vi "IterateShooter.vi"   [LabVIEW 2015]
uses:
  <vilib>/Rock Robotics/WPI/Solenoid/WPI_SolenoidValue.ctl
  <vilib>/Rock Robotics/WPI/Utilities/WPI_GetSetVariantRefNum.vi
  Robot Global Data.vi
  <vilib>/Rock Robotics/WPI/Solenoid/WPI_SolenoidSetEnum.vi
types:
  T1 = typedef "WPI_JoystickDevRef.ctl" = cluster{"Device":T2}
  T2 = typedef "WPI_JoystickDeviceEnum.ctl" = enum16{"USB 0", "USB 1", "USB 2", "USB 3", "USB 4", "USB 5"}
  T3 = typedef "constants.ctl" = cluster{"motorConstants":cluster{"leftDriveMotor":u8, "rightDriveMotor":u8, "climberWinch":T4, "shooterTopFlyWheel":T4, "shooterBottomFlyWheel":T4, "climberExtender":T4, "shooterIntakeWheel":u8, "Front Arm Motor":u8}, "arduinoInputChannel":cluster{"armAngleUp":i32, "intakeWheelSpinIn":i32, "winchUp":i32, "extenderUp":i32, "AimingAuto":i32, "extenderDown":i32, "FrontArmAxis":i32, "shooter up/down":i32}, "driveConstants":cluster{"firstIntervalPercent":dbl, "secondIntervalPercent":dbl, "thirdIntervalPercent":dbl}, "cRioInputChanels":cluster{"photoEye":i32, "limitExtender":i32}, "pneumaticsChannels":cluster{"angleSolenoid":T5, "shooterAnglerPneumaticForward":T5, "shooterAnglerPneumaticReverse":T5, "Pneumatics Control Module":u8}, "flyWheelConstants":cluster{"manualTopWheel":dbl, "manualBottomWheel":dbl, "autoFuncConst1":dbl, "autoFuncConst2":dbl, "autoFuncConst3":dbl, "autoFuncConst4":dbl, "Array":dbl[][]}}
  T4 = typedef "FPGA_DIOPWMChannel.ctl" = enum8{"PWM 0", "PWM 1", "PWM 2", "PWM 3", "PWM 4", "PWM 5", "PWM 6", "PWM 7", "PWM 8", "PWM 9", "PWM MXP 0", "PWM MXP 1", "PWM MXP 2", "PWM MXP 3", "PWM MXP 4", "PWM MXP 5", "PWM MXP 6", "PWM MXP 7", "PWM MXP 8", "PWM MXP 9", "Invalid"}
  T5 = typedef "WPI_SolenoidChannel.ctl" = enum8{"Solenoid 0", "Solenoid 1", "Solenoid 2", "Solenoid 3", "Solenoid 4", "Solenoid 5", "Solenoid 6", "Solenoid 7", "Invalid"}
  T6 = cluster{"Distance (ft)":dbl, "Center":cluster{dbl, dbl}, "Normalized Rect":cluster{"Numeric":dbl, "Numeric 2":dbl, "Numeric 3":dbl, "Numeric 5":dbl}}[]
  T7 = typedef "WPI_SolenoidValue.ctl" = enum16{"Off", "On", "Forward", "Reverse"}
  T8 = typedef "WPI_SolenoidDevRef.ctl" = cluster{"DevStatus":errorcluster, "Pneumatics Control Module":u8, "Forward Solenoid Channel":T5, "Reverse Solenoid Channel":T5}
  T9 = typedef "WPI_MotorControlDeviceRef.ctl" = cluster{"DeviceStatus":errorcluster, "Type":T10, "PWM":cluster{"PWM Channel":T4, "DeadBand":T11}, "CAN":cluster{"Device Number":u8, "Control Mode":T12, "Semaphore":T13, "Max Vout":dbl, "TalonSRX Control Mode":T14}, "Invert":bool}
  T10 = typedef "WPI_MotorControlType.ctl" = enum16{"PWM", "CAN", "CANTalonSRX"}
  T11 = typedef "WPI_PWMDeadband.ctl" = cluster{"Name":string, "maxPositivePwm":i32, "minPositivePwm":i32, "centerPwm":i32, "maxNegativePwm":i32, "minNegativePwm":i32, "angularRange":u16}
  T12 = typedef "WPI_CANJaguar_ControlMode.ctl" = enum8{"Percent VBus", "Current", "Speed", "Position", "Voltage"}
  T13 = typedef "Semaphore RefNum" = refnum<k1>
  T14 = typedef "WPI_CANTalonSRX_APIControlMode.ctl" = enum8{"Percent VBus", "Speed", "Position", "Slave", "Unchanged / Invalid", "Voltage Compensation", "Current", "Motion Profile"}
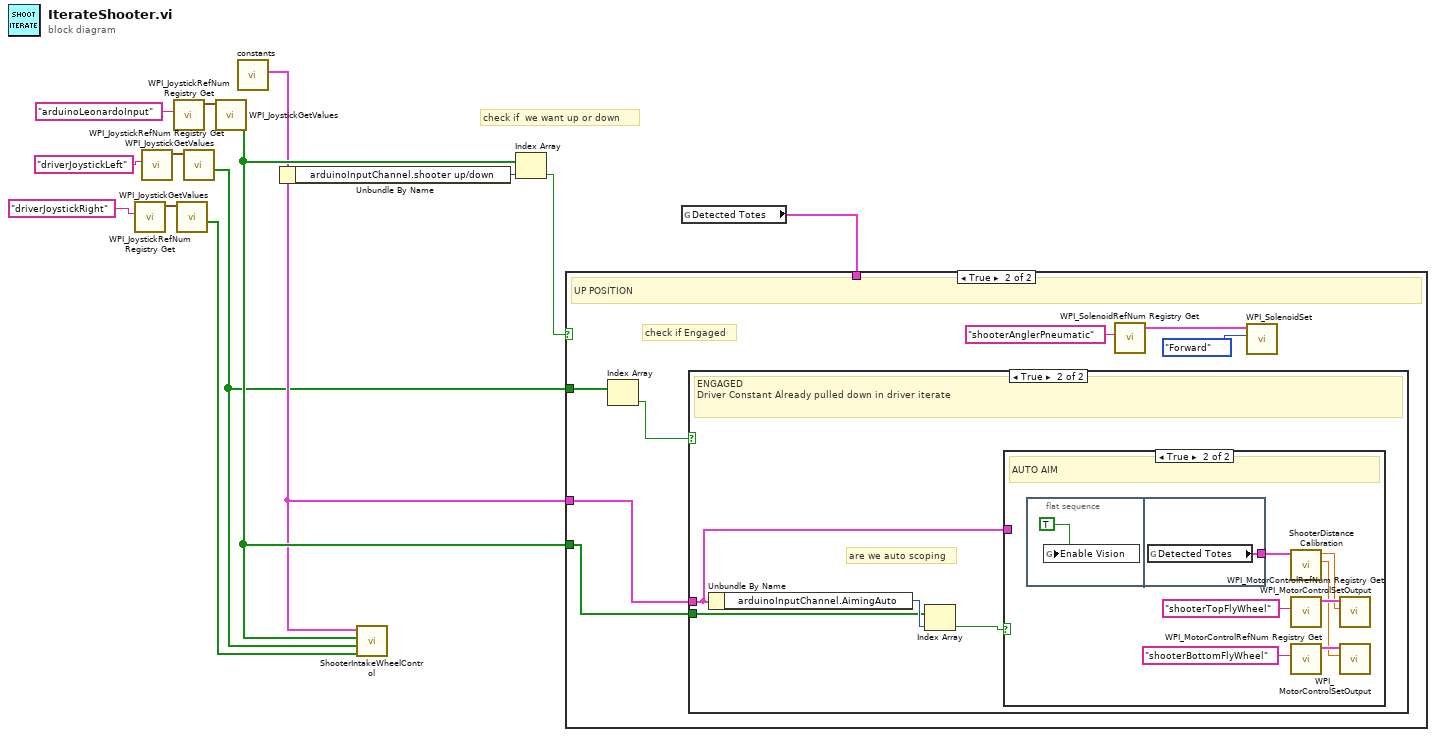
[diagram p0: block diagram]
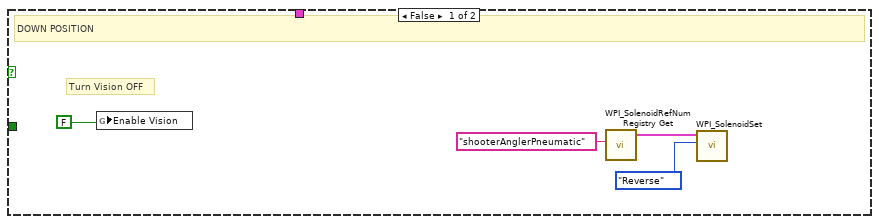
[diagram p2: hidden frame]
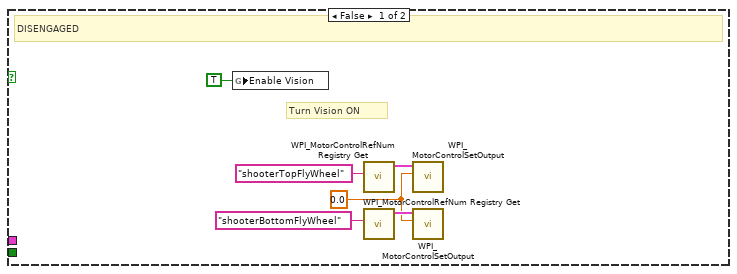
[diagram p3: hidden frame]
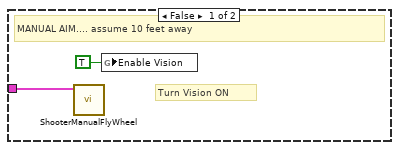
[diagram p4: hidden frame]
diagram:
  # "check if  we want up or down"
  n1 = call <vilib>:"WPI_JoystickRefNum Registry Get.vi"("refnum name"="driverJoystickRight") -> ("JoystickDevRef"=w8:T1)  [unwired: 9 in, 1 out]
  n2 = call <vilib>:"WPI_JoystickRefNum Registry Get.vi"("refnum name"="driverJoystickLeft") -> ("JoystickDevRef"=w9:T1)  [unwired: 9 in, 1 out]
  n3 = call <vilib>:"WPI_JoystickRefNum Registry Get.vi"("refnum name"="arduinoLeonardoInput") -> ("JoystickDevRef"=w12:T1)  [unwired: 9 in, 1 out]
  n4 = call <vilib>:"WPI_JoystickGetValues.vi"("JoystickDevRef"=w8) -> ("Buttons"=w4:bool[])  [unwired: 6 in, 4 out]
  n5 = call <vilib>:"WPI_JoystickGetValues.vi"("JoystickDevRef"=w9) -> ("Buttons"=w5:bool[])  [unwired: 6 in, 4 out]
  n6 = call <vilib>:"WPI_JoystickGetValues.vi"("JoystickDevRef"=w12) -> ("Buttons"=w7:bool[])  [unwired: 6 in, 4 out]
  n7 = call "constants.vi"() -> (2:w6:T3)  [unwired: 11 in]
  n8 = Unbundle By Name(w6) -> ("arduinoInputChannel.shooter up/down"=w11:i32)
  n9 = call "ShooterIntakeWheelControl.vi"("Constants"=w6, "leonardoJoystick"=w7, "driverJoystickLeft"=w5, "driverJoystickRight"=w4) -> ()  [unwired: 6 in]
  n10 = Index Array(array=w7, index=w11) -> (element=w10:bool)
  n11 = global read "Robot Global Data.vi" "Detected Totes"() -> (w1:T6)
  n12 = case shown="True" w10 {
    tunnel: w7 -> [_ w22]
    tunnel: w6 -> [_ w23]
    tunnel: w5 -> [_ w21]
    tunnel: w1 -> [_ _]
    frame False {
      # "Turn Vision OFF"
      # "DOWN POSITION"
      n13 = global write "Robot Global Data.vi" "Enable Vision"(FALSE ("Enable Vision")) -> ()
      n14 = call <vilib>:"WPI_SolenoidRefNum Registry Get.vi"("refnum name"="shooterAnglerPneumatic") -> ("SolenoidDevRef"=w15:T8)  [unwired: 9 in, 1 out]
      n15 = call-poly <vilib>:"WPI_SolenoidSet.vi"("Value"=WPI_SolenoidValue."Reverse", "SolenoidDevRef"=w15) -> ()  [unwired: 8 in, 2 out]
    }
    frame True {
      # "check if Engaged"
      # "UP POSITION"
      n16 = Index Array(array=w21) -> (element=w24:bool)  [unwired: 1 in]
      n17 = case shown="True" w24 {
        tunnel: w23 -> [_ w31]
        tunnel: w22 -> [_ w32]
        frame False {
          w26 = 0.0 ("Output")
          # "Turn Vision ON"
          # "DISENGAGED"
          n18 = global write "Robot Global Data.vi" "Enable Vision"(TRUE ("Enable Vision")) -> ()
          n19 = call <vilib>:"WPI_MotorControlRefNum Registry Get.vi"("refnum name"="shooterTopFlyWheel") -> ("MotorControlDevRef"=w25:T9)  [unwired: 9 in, 1 out]
          n20 = call <vilib>:"WPI_MotorControlRefNum Registry Get.vi"("refnum name"="shooterBottomFlyWheel") -> ("MotorControlDevRef"=w29:T9)  [unwired: 9 in, 1 out]
          n21 = call <vilib>:"WPI_MotorControlSetOutput.vi"("Output"=w26, "MotorControlDevRef"=w25) -> ()  [unwired: 7 in, 3 out]
          n22 = call <vilib>:"WPI_MotorControlSetOutput.vi"("Output"=w26, "MotorControlDevRef"=w29) -> ()  [unwired: 7 in, 3 out]
        }
        frame True {
          # "are we auto scoping"
          # "ENGAGED\nDriver Constant Already pulled down in driver iterate"
          n23 = Unbundle By Name(w31) -> ("arduinoInputChannel.AimingAuto"=w34:i32)
          n24 = Index Array(array=w32, index=w34) -> (element=w33:bool)
          n25 = case shown="True" w33 {
            tunnel: w31 -> [w35 _]
            frame False {
              # "Turn Vision ON"
              # "MANUAL AIM.... assume 10 feet away"
              n26 = call "ShooterManualFlyWheel.vi"("Cluster"=w35) -> ()  [unwired: 11 in]
              n27 = global write "Robot Global Data.vi" "Enable Vision"(TRUE ("Enable Vision")) -> ()
            }
            frame True {
              # "AUTO AIM"
              n28 = flat-sequence {
                tunnel: [w45] -> w39
                frame #0 {
                  n29 = global write "Robot Global Data.vi" "Enable Vision"(TRUE ("Enable Vision")) -> ()
                }
                frame #1 {
                  n30 = global read "Robot Global Data.vi" "Detected Totes"() -> (w45:T6)
                }
              }
              n31 = call "ShooterDistanceCalibration.vi"("Detected Totes"=w39) -> ("bottomFlyWheelConstant"=w37:dbl, "TopFlyWheelConstant"=w38:dbl)  [unwired: 9 in]
              n32 = call <vilib>:"WPI_MotorControlRefNum Registry Get.vi"("refnum name"="shooterTopFlyWheel") -> ("MotorControlDevRef"=w41:T9)  [unwired: 9 in, 1 out]
              n33 = call <vilib>:"WPI_MotorControlRefNum Registry Get.vi"("refnum name"="shooterBottomFlyWheel") -> ("MotorControlDevRef"=w43:T9)  [unwired: 9 in, 1 out]
              n34 = call <vilib>:"WPI_MotorControlSetOutput.vi"("Output"=w38, "MotorControlDevRef"=w41) -> ()  [unwired: 7 in, 3 out]
              n35 = call <vilib>:"WPI_MotorControlSetOutput.vi"("Output"=w37, "MotorControlDevRef"=w43) -> ()  [unwired: 7 in, 3 out]
            }
          }
        }
      }
      n36 = call <vilib>:"WPI_SolenoidRefNum Registry Get.vi"("refnum name"="shooterAnglerPneumatic") -> ("SolenoidDevRef"=w19:T8)  [unwired: 9 in, 1 out]
      n37 = call-poly <vilib>:"WPI_SolenoidSet.vi"("Value"=WPI_SolenoidValue."Forward", "SolenoidDevRef"=w19) -> ()  [unwired: 8 in, 2 out]
    }
  }
